vi "SeparateCmd_3.vi"(8 "connection ID":refnum<k5>, 9 "CmdID":string, 11 "command received":string) -> (1 "CmdInProgress":T1(array[cluster]), 3 "Client Name":string)   [LabVIEW 2011]
uses:
  <vilib>/regexp/Match Regular Expression.xnode
panel:
  out "Command":string
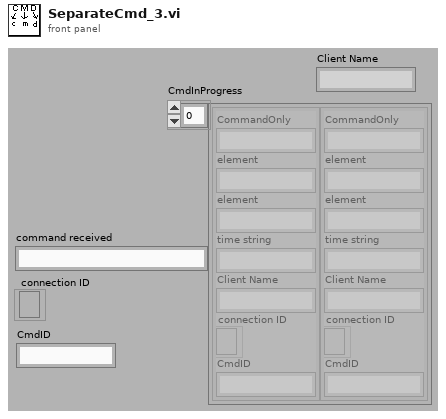
[diagram p1: front panel]
types:
  T1 = cluster{"CommandOnly":string, "element":string, "element":string, "time string":string, "Client Name":string, "connection ID":refnum<k5>, "CmdID":string}[]
  T2 = cluster{"CommandOnly":string, "element":string, "element":string, "time string":string, "Client Name":string, "connection ID":refnum<k5>, "CmdID":string}
  T3 = cluster{"before match":string, "element":string, "element":string, string, string, "connection ID":refnum<k5>, "CmdID":string}
  T4 = cluster{string, "element":string, "element":string, string, string, "connection ID":refnum<k5>, "CmdID":string}
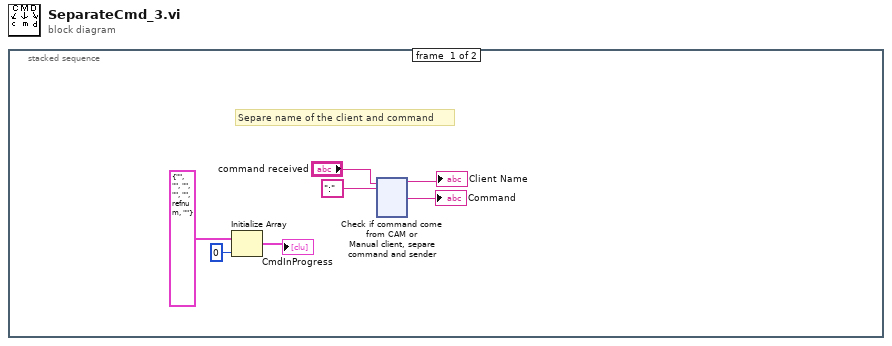
[diagram p0: block diagram]
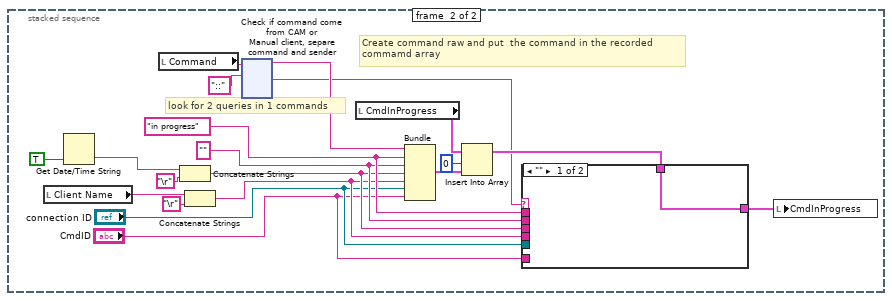
[diagram p2: hidden frame]
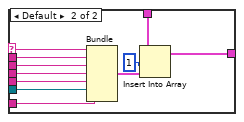
[diagram p3: hidden frame]
diagram:
  n1 = stacked-sequence {
    frame #0 {
      # "Separe name of the client and command"
      n2 = Initialize Array(T2 {"CommandOnly"="", "element"="", "element"="", "time string"="", "Client Name"="", "connection ID"=refnum, "CmdID"=""} ("CmdInProgress"), 0 ("dimension size")) -> (→"CmdInProgress":T1)
      n3 = xnode ("Check if command come from CAM or\nManual client, separe command and sender")("input string"="command received", "regular expression"=":") -> ("before match"=→"Client Name":string, "after match"=→"Command":string)  [unwired: 2 in, 5 out]
    }
    frame #1 {
      w132 = "" ("element")
      w133 = "in progress" ("element")
      # "look for 2 queries in 1 commands"
      # "Create command raw and put  the command in the recorded\ncommamd array"
      n4 = local read "Client Name"() -> (w136:string)
      n5 = Get Date/Time String(want seconds? (F)=TRUE) -> (time string=w135:string)  [unwired: 1 in, 2 out]
      n6 = local read "Command"() -> (w127:string)
      n7 = Concatenate Strings(w135, "\r") -> (w131:string)
      n8 = Concatenate Strings(w136, "\r") -> (w130:string)
      n9 = xnode ("Check if command come from CAM or\nManual client, separe command and sender")("input string"=w127, "regular expression"="::") -> ("before match"=w120:string, "after match"=w119:string)  [unwired: 2 in, 5 out]
      n10 = local read "CmdInProgress"() -> (w125:T1)
      n11 = Bundle("before match"=w120, "element"=w133, "element"=w132, w131, w130, "connection ID"="connection ID", "CmdID"="CmdID") -> (w123:T3)  [unwired: 1 out]
      n12 = Insert Into Array(array=w125, index=0, new element=w123) -> (w122:T1)
      n13 = case shown="\"\"" w119 {
        selector: w119 -> [_ w140]
        tunnel: w133 -> [_ w150]
        tunnel: w132 -> [_ w149]
        tunnel: w131 -> [_ w148]
        tunnel: w122 -> [w139 w147]
        tunnel: [w139 w146] -> w126
        tunnel: w130 -> [_ w144]
        tunnel: "connection ID" -> [_ w143]
        tunnel: "CmdID" -> [_ w142]
        frame "" {
        }
        frame Default {
          n14 = Bundle(w140, "element"=w150, "element"=w149, w148, w144, "connection ID"=w143, "CmdID"=w142) -> (w145:T4)  [unwired: 1 out]
          n15 = Insert Into Array(array=w147, index=1, new element=w145) -> (w146:T1)
        }
      }
      n16 = local write "CmdInProgress"(w126) -> ()
    }
  }
